vi "GetFiles.vi"(8 "error in (no error)":errorcluster, 11 "Python":T1) -> (0 "error out":errorcluster, 3 "all files":string[](array[string]))   [LabVIEW 2021]
uses:
  PythonCtrl.ctl
  Processors.ctl
  Comm_Global.vi
panel:
  out "Console":string
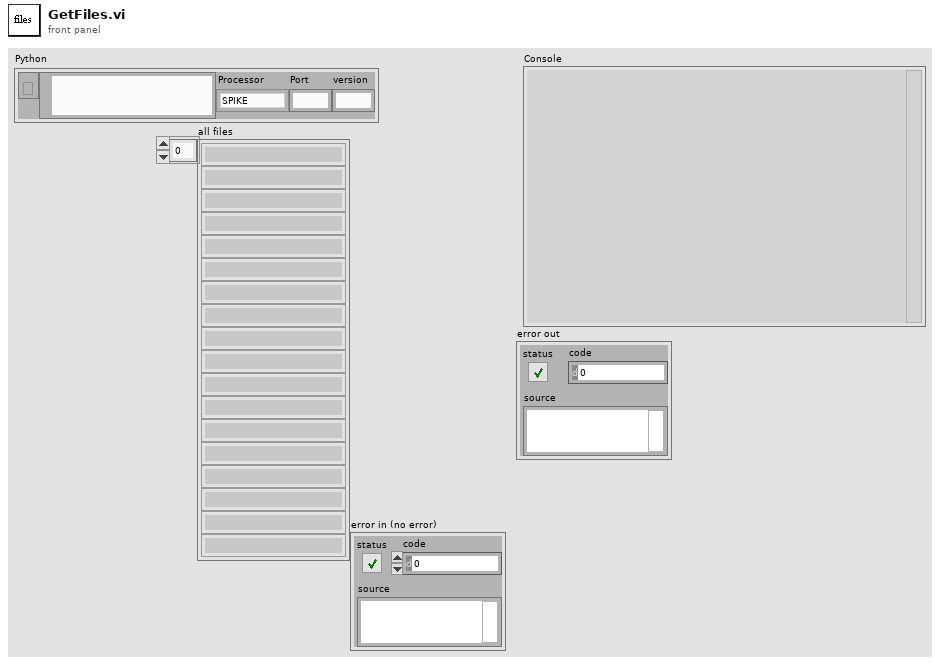
[diagram p1: front panel]
types:
  T1 = typedef "PythonCtrl.ctl" = cluster{"session":refnum<k35>, "PyPath":path, "Processor":T2, "Port":string, "version":string}
  T2 = typedef "Processors.ctl" = enum16{"SPIKE", "Pi", "Pi_ssh", "OpenMV", "Dunio"}
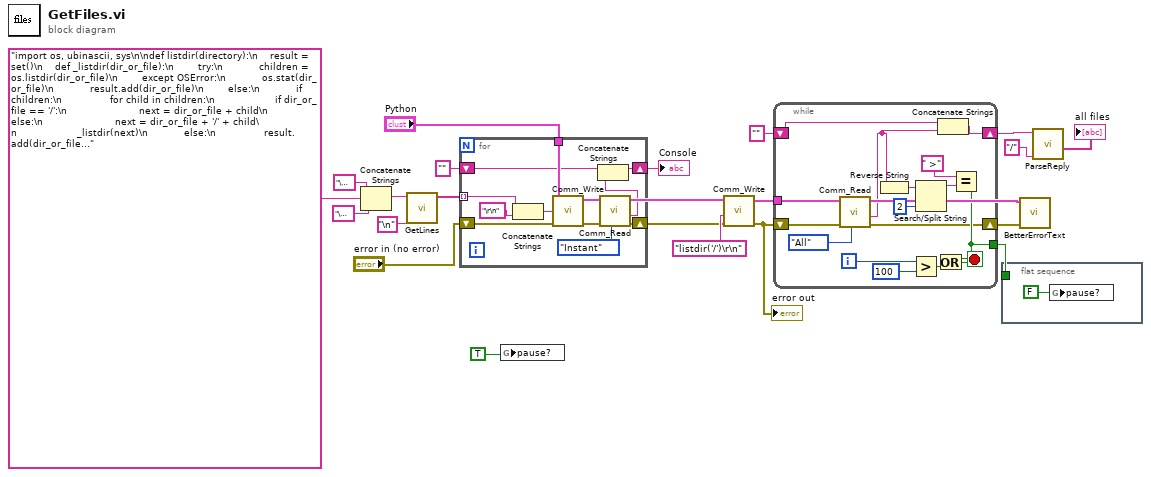
[diagram p0: block diagram]
diagram:
  n1 = Concatenate Strings("\u0005" ("string"), "import os, ubinascii, sys\n\ndef listdir(directory):\n    result = set()\n    def _listdir(dir_or_file):\n        try:\n            children = os.listdir(dir_or_file)\n        except OSError:\n            os.stat(dir_or_file)\n            result.add(dir_or_file)\n        else:\n            if children:\n                for child in children:\n                    if dir_or_file == '/':\n                        next = dir_or_file + child\n                    else:\n                        next = dir_or_file + '/' + child\n                    _listdir(next)\n            else:\n                result.add(dir_or_file)\n    _listdir(directory)\n    return sorted(result)\n\ndef readfile(file):\n    with open(file, 'rb') as infile:\n        while True:\n            result = infile.read(32)\n            if result == b'':\n                break\n            len = sys.stdout.write(ubinascii.hexlify(result))\n\n" ("function name"), "\u0004" ("string")) -> (w10:string)
  n2 = call "GetLines.vi"("delimiter"="\n" ("function name"), "String"=w10) -> ("Array"=w7:string[])  [unwired: 9 in]
  n3 = for {
    tunnel: "Python" -> [w27]
    shift-right: [w28] -> w11
    shift-left: "error in (no error)" -> [w31]
    tunnel: w7 -> [w26] mode=indexing
    shift-right: [w22] -> w8
    shift-left: "" -> [w24]
    n4 = Concatenate Strings(w26, "\r\n" ("function name")) -> (w25:string)
    n5 = call "Comm_Write.vi"("error in (no error)"=w31, "Text to write"=w25, "Python"=w27) -> ("error out"=w30:errorcluster)  [unwired: 7 in, 1 out]
    n6 = call "Comm_Read.vi"("Task"=enum16{"Instant", "All", "AllFast", "Params"}."Instant", "error in (no error)"=w30, "Python"=w27) -> ("error out"=w28:errorcluster, "Text read"=w23:string)  [unwired: 7 in]
    n7 = Concatenate Strings(w24, w23) -> (w22:string)
  }
  "Console" <- w8
  n8 = global write "Comm_Global.vi" "pause?"(TRUE ("pause?")) -> ()
  n9 = call "Comm_Write.vi"("error in (no error)"=w11, "Text to write"="listdir('/')\r\n" ("function name"), "Python"="Python") -> ("error out"=w16:errorcluster)  [unwired: 7 in, 1 out]
  "error out" <- w16
  n10 = while {
    tunnel: "Python" -> [w46]
    tunnel: [w36] -> w5
    shift-right: [w33] -> w18
    shift-left: "" ("Text read") -> [w35]
    shift-right: [w32] -> w2
    shift-left: w16 -> [w45]
    i -> [w44]
    stop <- w41 stop-if-true
    n11 = call "Comm_Read.vi"("Task"=enum16{"Instant", "All", "AllFast"}."All", "error in (no error)"=w45, "Python"=w46) -> ("error out"=w32:errorcluster, "Text read"=w34:string)  [unwired: 7 in]
    n12 = Reverse String(1:w34) -> (0:w40:string)
    n13 = Greater?(x=w44, y=100) -> (0:w42:bool)
    n14 = Search/Split String(string=w40, offset (0)=2) -> (substring before match=w38:string)  [unwired: 1 in, 2 out]
    n15 = Concatenate Strings(w35, w34) -> (w33:string)
    n16 = Equal?(x=" >", y=w38) -> (x = y?=w36:bool)
    n17 = Or(x=w36, y=w42) -> (x .or. y?=w41:bool)
  }
  n18 = flat-sequence {
    tunnel: w5 -> [_]
    frame #0 {
      n19 = global write "Comm_Global.vi" "pause?"(FALSE ("pause?")) -> ()
    }
  }
  n20 = call "BetterErrorText.vi"("error in (no error)"=w2, "Python"="Python") -> ()  [unwired: 8 in, 2 out]
  n21 = call "ParseReply.vi"("Parent"="/" ("trimmed string"), "Console"=w18) -> ("PythonFiles"=→"all files":string[])  [unwired: 7 in, 2 out]
